vi "Commit Properties for Devices.vi"(0 "session in":refnum<k21>, 5 "devices":refnum<k21>="$DefaultDevices", 11 "error in (no error)":errorcluster) -> (4 "session out":refnum<k21>, 15 "error out":errorcluster)   [LabVIEW 2020, in "SLSC.lvlib"]
doc: "Commits all device or physical channels properties with pending changes to hardware, for the specified device(s) and the physical channels that they contain. If you set a property multiple times between commits, only the last value will be committed."
uses:
  <vilib>/SLSC/SLSC.lvlib
  nislsclvapi.dll
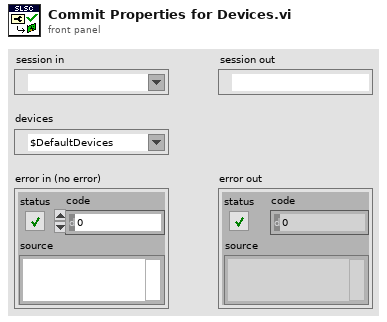
[diagram p1: front panel]
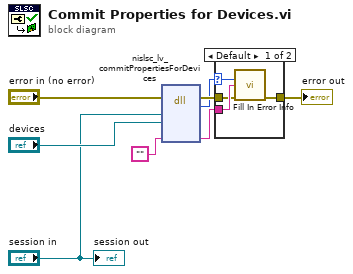
[diagram p0: block diagram]
diagram:
  n1 = dll-call lib="nislsclvapi.*" fn="nislsc_lv_commitPropertiesForDevices"(error in="error in (no error)", "session"="session in", "devices"="devices", "extendedErrorInfo"="") -> (error out=w6:errorcluster, "return type"=w5:i32, "extendedErrorInfo"=w7:string)  [unwired: 6 in, 1 out]
  n2 = case shown="Default" w5 {
    selector: w5 -> [w12 _]
    tunnel: w7 -> [w11 _]
    tunnel: w6 -> [w10 w13]
    tunnel: [w9 w13] -> w4
    frame Default {
      n3 = call <vilib>:"Fill In Error Info.vi"("status code"=w12, "extended error info"=w11, "error in"=w10) -> ("error out"=w9:errorcluster)  [unwired: 12 in]
    }
    frame 0 {
    }
  }
  "error out" <- w4
  "session out" <- "session in"
